vi "splitControl.vi"(11 "driveStatus":bool) -> (1 "JoystickDevRef 2":T1, 2 "JoystickDevRef":T1)   [LabVIEW 2016]
uses:
  <vilib>/Rock Robotics/WPI/Joystick/WPI_JoystickDevRef.ctl
  <vilib>/Rock Robotics/WPI/Joystick/WPI_JoystickDeviceEnum.ctl
  <vilib>/Rock Robotics/WPI/Utilities/WPI_GetSetVariantRefNum.vi
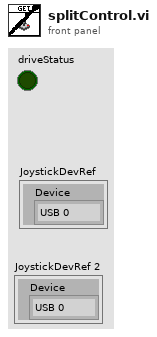
[diagram p1: front panel]
types:
  T1 = typedef "WPI_JoystickDevRef.ctl" = cluster{"Device":T2}
  T2 = typedef "WPI_JoystickDeviceEnum.ctl" = enum16{"USB 0", "USB 1", "USB 2", "USB 3", "USB 4", "USB 5"}
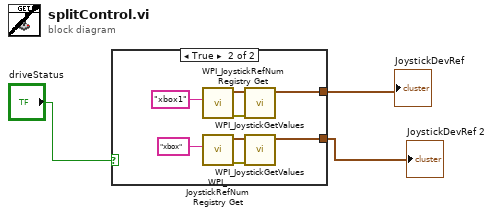
[diagram p0: block diagram]
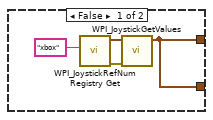
[diagram p2: hidden frame]
diagram:
  n1 = case shown="True" "driveStatus" {
    tunnel: [w4 w12] -> w1
    tunnel: [w4 w8] -> w2
    frame False {
      n2 = call <vilib>:"WPI_JoystickRefNum Registry Get.vi"("refnum name"="xbox") -> ("error out"=w6:errorcluster, "JoystickDevRef"=w5:T1)  [unwired: 9 in]
      n3 = call <vilib>:"WPI_JoystickGetValues.vi"("error in (no error)"=w6, "JoystickDevRef"=w5) -> ("JoystickDevRef"=w4:T1)  [unwired: 5 in, 4 out]
    }
    frame True {
      n4 = call <vilib>:"WPI_JoystickRefNum Registry Get.vi"("refnum name"="xbox1") -> ("error out"=w10:errorcluster, "JoystickDevRef"=w9:T1)  [unwired: 9 in]
      n5 = call <vilib>:"WPI_JoystickRefNum Registry Get.vi"("refnum name"="xbox") -> ("error out"=w14:errorcluster, "JoystickDevRef"=w13:T1)  [unwired: 9 in]
      n6 = call <vilib>:"WPI_JoystickGetValues.vi"("error in (no error)"=w10, "JoystickDevRef"=w9) -> ("JoystickDevRef"=w8:T1)  [unwired: 5 in, 4 out]
      n7 = call <vilib>:"WPI_JoystickGetValues.vi"("error in (no error)"=w14, "JoystickDevRef"=w13) -> ("JoystickDevRef"=w12:T1)  [unwired: 5 in, 4 out]
    }
  }
  "JoystickDevRef" <- w2
  "JoystickDevRef 2" <- w1
